vi "Main.vi"() -> ()   [LabVIEW 2019, in "Template Server.lvlib" / "Template Server.lvclass"]
uses:
  Template Server.lvclass
  typeDefs/Server State Data.ctl
panel:
  out "Listening Port":i32
  in  "Stop":bool
  in  "Enable Async Mode":bool
  in  "Server Address":string="0.0.0.0:50051"
  in  "Server Certificate File (.crt)":path
  in  "Server Key File (.key)":path
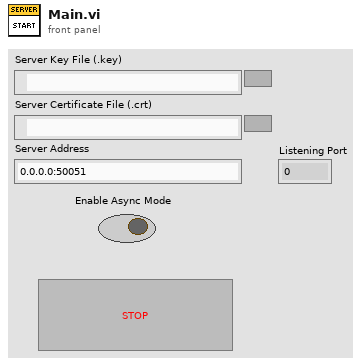
[diagram p1: front panel]
types:
  T1 = typedef "Template Server.lvlib/Template Server.lvclass/Server State Data.ctl" = cluster{"Data":string}
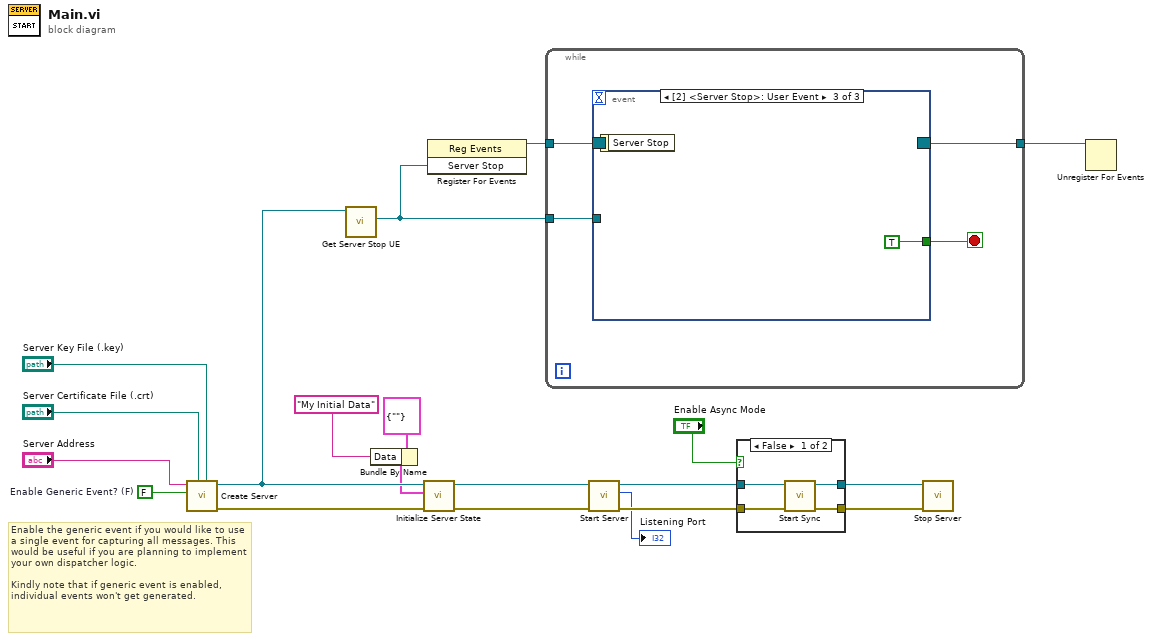
[diagram p0: block diagram]
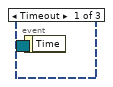
[diagram p2: hidden frame]
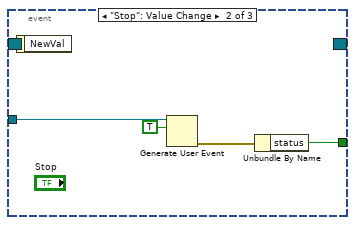
[diagram p3: hidden frame]
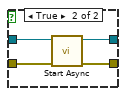
[diagram p4: hidden frame]
diagram:
  w1 = FALSE  # Enable Generic Event? (F)
  # "Enable the generic event if you would like to use a single event for capturing all messages. This would be useful if you are planning to implement your own dispatcher logic.\n\nKindly note that if generic event is enabled, individual events won't get generated."
  n1 = call "Create Server.vi"("Server Key File (.key)"="Server Key File (.key)", "Server Certificate File (.crt)"="Server Certificate File (.crt)", "Enable Generic Event? (F)"=w1, "Server Address"="Server Address") -> ("error out"=w9:errorcluster, "gRPC Server out"=w6:refnum<class "Template Server.lvclass">)  [unwired: 6 in]
  n2 = call "Get Server Stop UE.vi"("OOP Server in"=w6) -> ("Server Stop"=w10:refnum<user-event>)  [unwired: 9 in, 1 out]
  n3 = Bundle By Name(cluster=T1 {"Data"=""} ("Initial State"), "Data"="My Initial Data") -> (w4:T1)
  n4 = call "Initialize Server State.vi"("error in (no error)"=w9, "Initial State"=w4, "gRPC Server in"=w6) -> ("error out"=w8:errorcluster, "gRPC Server out"=w7:refnum<class "Template Server.lvclass">)  [unwired: 7 in]
  n5 = register-events(w10) -> (reference out=w12:refnum<event-registration>)  [unwired: 2 in, 1 out]
  n6 = while {
    tunnel: w10 -> [w24]
    tunnel: w12 -> [w23]
    tunnel: [w21] -> w11
    stop <- w22 stop-if-true
    n7 = event shown="[2] <Server Stop>: User Event" {
      selector: w23 -> [_ _ _]
      dyn-events: [_ _ _] -> w21
      timeout: _ -> [_ _ _]
      tunnel: w24 -> [_ w28 _]
      tunnel: [_ w25 TRUE] -> w22
      event Timeout {
        n8 = event-data() -> ()  [unwired: 1 in, 1 out]
      }
      event "Stop": Value Change {
        n9 = event-data() -> ()  [unwired: 1 in, 1 out]
        n10 = Generate User Event(user event=w28, event data cluster=TRUE ("event data")) -> (error out=w26:errorcluster)  [unwired: 2 in, 1 out]
        n11 = Unbundle By Name(w26) -> ("status"=w25:bool)
      }
      event User Event {
        n12 = event-data() -> ()  [unwired: 1 in, 1 out]
      }
    }
  }
  n13 = call "Start Server.vi"("error in (no error)"=w8, "gRPC Server in"=w7) -> ("error out"=w20:errorcluster, "Listening Port"=→"Listening Port":i32, "gRPC Server out"=w19:refnum<class "Template Server.lvclass">)  [unwired: 7 in]
  n14 = case shown="False" "Enable Async Mode" {
    tunnel: w20 -> [w33 w37]
    tunnel: w19 -> [w32 w36]
    tunnel: [w31 w34] -> w18
    tunnel: [w30 w35] -> w17
    frame False {
      n15 = call "Start Sync.vi"("error in (no error)"=w33, "gRPC Server in"=w32) -> ("error out"=w31:errorcluster, "gRPC Server out"=w30:refnum<class "Template Server.lvclass">)  [unwired: 8 in]
    }
    frame True {
      n16 = call "Start Async.vi"("error in (no error)"=w37, "gRPC Server in"=w36) -> ("error out"=w34:errorcluster, "gRPC Server out"=w35:refnum<class "Template Server.lvclass">)  [unwired: 8 in]
    }
  }
  n17 = call "Stop Server.vi"("error in (no error)"=w18, "gRPC Server in"=w17) -> ()  [unwired: 9 in, 1 out]
  n18 = Unregister For Events(event registration refnum=w11) -> ()  [unwired: 1 in, 1 out]
